vi "loadMT2FinalBin100Yld.vi"() -> ()   [LabVIEW 2012]
uses:
  <vilib>/addons/database/Auxilliary.llb/DB Tools Cursor Type.ctl
  <vilib>/addons/database/Connection.llb/DB Tools Open Connec (Path).vi
  <vilib>/addons/database/Connection.llb/Conn Execute.vi
  <vilib>/addons/database/Recordset.llb/Rec Fetch Recordset Data (R).vi
  <vilib>/addons/database/Recordset.llb/Rec Destroy - Connection.vi
  <vilib>/addons/database/_DB Variant To Data/Database Variant To Data.xnode
  <vilib>/addons/database/NI_Database_API.lvlib
panel:
  out "recordset data":variant[][](array[variant])
  out "data":string
  out "error out":errorcluster
  out "concatenated string":string
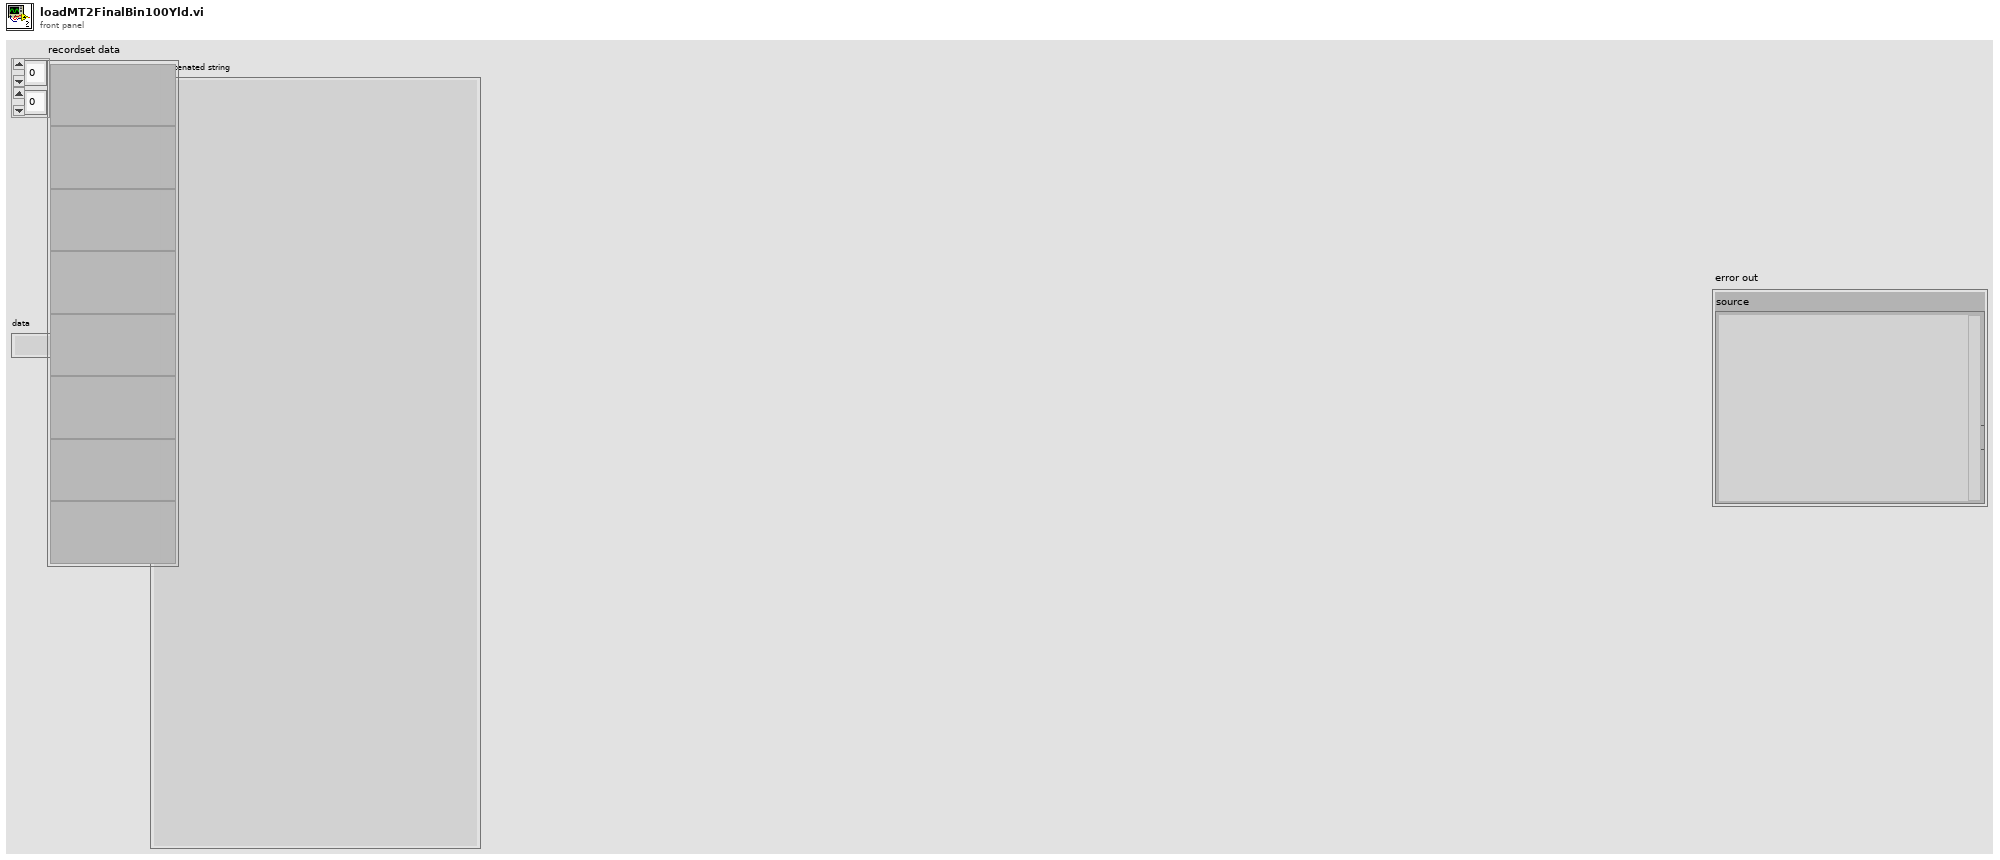
[diagram p1: front panel]
types:
  T1 = typedef "NI_Database_API.lvlib/DB Tools Cursor Type.ctl" = enum16{"forward-only", "keyset", "dynamic", "static"}
  T2 = typedef "NI_Database_API.lvlib/Conn ObjectReference.ctl" = refnum<k1>
  T3 = typedef "NI_Database_API.lvlib/Rec ObjectReference.ctl" = refnum<k1>
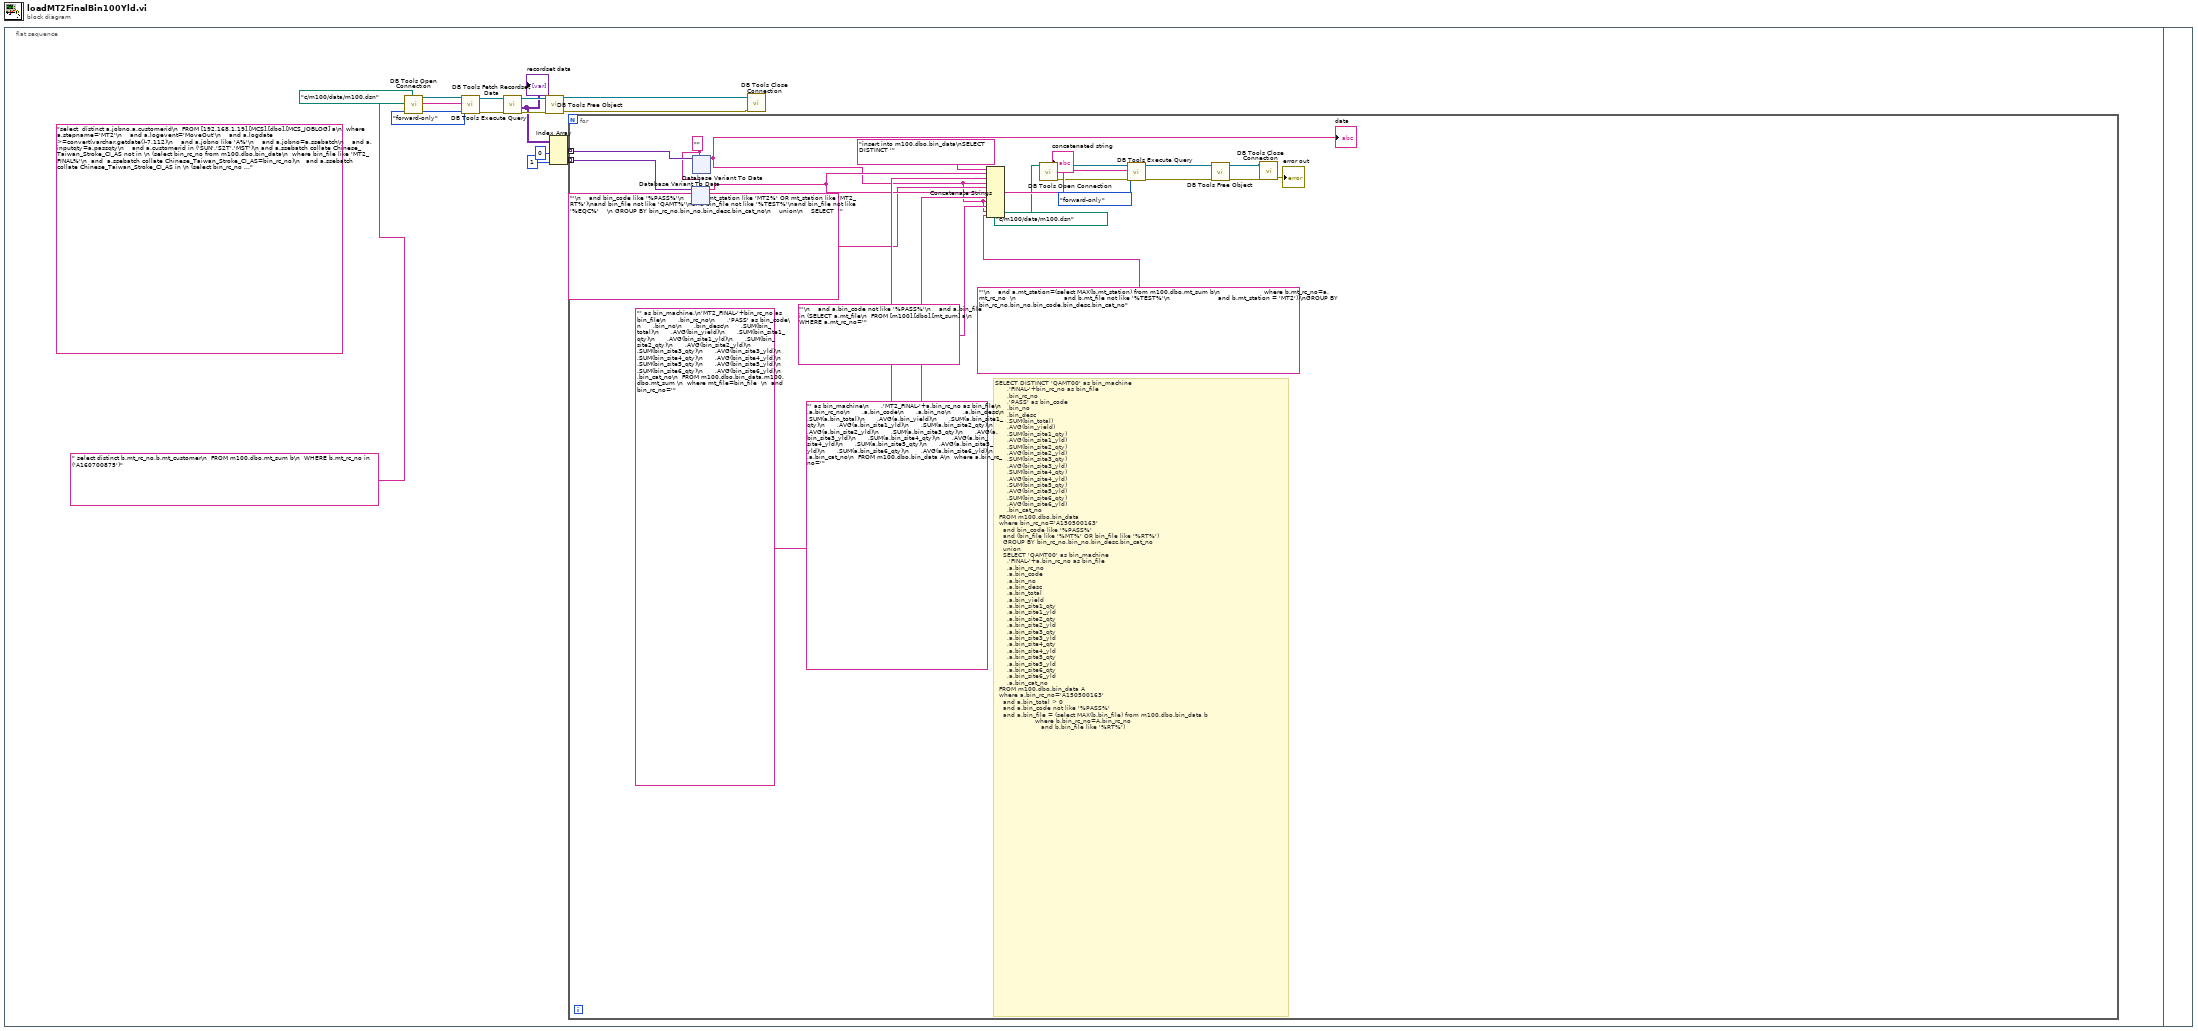
[diagram p0: block diagram]
diagram:
  n1 = flat-sequence {
    frame #0 {
      (unwired) "select  distinct a.jobno,a.customerid\n  FROM [192.168.1.19].[MCS].[dbo].[MCS_JOBLOG] a\n  where  a.stepname='MT2'\n    and a.logevent='MoveOut'\n    and a.logdate >=convert(varchar,getdate()-7,112)\n    and a.jobno like 'A%'\n    and a.jobno=a.ssebatch\n    and a.inputqty=a.passqty\n    and a.customerid in ('SUN','S2T','MST')\n and a.ssebatch collate Chinese_Taiwan_Stroke_CI_AS not in \n (select bin_rc_no from m100.dbo.bin_data\n  where bin_file like 'MT2_FINAL%'\n  and  a.ssebatch collate Chinese_Taiwan_Stroke_CI_AS=bin_rc_no)\n   and a.ssebatch collate Chinese_Taiwan_Stroke_CI_AS in \n (select bin_rc_no from m100.dbo.bin_data\n  where bin_file like '%MT2%'\n  and  a.ssebatch collate Chinese_Taiwan_Stroke_CI_AS=bin_rc_no)\n " ("SQL query")
      n2 = call-poly <vilib>:"DB Tools Open Connection.vi"("connection information"=path "c:/m100/data/m100.dsn") -> ("error out"=w13:errorcluster, "connection reference"=w16:T2)  [unwired: 7 in]
      n3 = call-poly <vilib>:"DB Tools Execute Query.vi"("error in (no error)"=w13, "cursor type"=DB_Tools_Cursor_Type."forward-only", "SQL query"=" select distinct b.mt_rc_no,b.mt_customer\n  FROM m100.dbo.mt_sum b\n  WHERE b.mt_rc_no in ('A160700875')", "connection reference"=w16) -> ("error out"=w12:errorcluster, "recordset reference"=w15:T3)  [unwired: 4 in]
      n4 = call-poly <vilib>:"DB Tools Fetch Recordset Data.vi"("error in (no error)"=w12, "recordset reference"=w15) -> ("error out"=w11:errorcluster, "recordset data"=w8:variant[][], "recordset reference out"=w14:T3)  [unwired: 3 in]
      "recordset data" <- w8
      n5 = call-poly <vilib>:"DB Tools Free Object.vi"("error in (no error)"=w11, "recordset reference"=w14) -> ("error out"=w4:errorcluster, "connection reference"=w5:T2)  [unwired: 8 in]
      n6 = Index Array(array=w8, index (col) #1=0 ("disabled index (col)"), index (col) #2=1 ("index (col)")) -> (element #1=w6:variant[], element #2=w2:variant[])  [unwired: 2 in]
      n7 = for {
        tunnel: w6 -> [w37] mode=indexing
        tunnel: w2 -> [w25] mode=indexing
        w24 = ""
        # "SELECT DISTINCT 'QAMT00' as bin_machine\n      ,'FINAL-'+bin_rc_no as bin_file\n      ,bin_rc_no\n      ,'PASS' as bin_code\n      ,bin_no\n      ,bin_desc\n      ,SUM(bin_total)\n      ,AVG(bin_yield)\n      ,SUM(bin_site1_qty)\n      ,AVG(bin_site1_yld)\n      ,SUM(bin_site2_qty)\n      ,AVG(bin_site2_yld)\n      ,SUM(bin_site3_qty)\n      ,AVG(bin_site3_yld)\n      ,SUM(bin_site4_qty)\n      ,AVG(bin_site4_yld)\n      ,SUM(bin_site5_qty)\n      ,AVG(bin_site5_yld)\n      ,SUM(bin_site6_qty)\n      ,AVG(bin_site6_yld)\n      ,bin_cat_no\n  FROM m100.dbo.bin_data\n  where bin_rc_no='A150500163'\n    and bin_code like '%PASS%'\n    and (bin_file like '%MT%' OR bin_file like '%RT%')\n    GROUP BY bin_rc_no,bin_no,bin_desc,bin_cat_no\n    union\n    SELECT 'QAMT00' as bin_machine\n      ,'FINAL-'+a.bin_rc_no as bin_file\n      ,a.bin_rc_no\n      ,a.bin_code\n      ,a.bin_no\n      ,a.bin_desc\n      ,a.bin_total\n      ,a.bin_yield\n      ,a.bin_site1_qty\n      ,a.bin_site1_yld\n      ,a.bin_site2_qty\n      ,a.bin_site2_yld\n      ,a.bin_site3_qty\n      ,a.bin_site3_yld\n      ,a.bin_site4_qty\n      ,a.bin_site4_yld\n      ,a.bin_site5_qty\n      ,a.bin_site5_yld\n      ,a.bin_site6_qty\n      ,a.bin_site6_yld\n      ,a.bin_cat_no\n  FROM m100.dbo.bin_data A\n  where a.bin_rc_no='A150500163'\n    and a.bin_total > 0\n    and a.bin_code not like '%PASS%'\n    and a.bin_file = (select MAX(b.bin_file) from m100.dbo.bin_data b\n                    where b.bin_rc_no=A.bin_rc_no\n                       and b.bin_file like '%RT%')"
        n8 = xnode "Database Variant To Data"("database variant"=w25, "type"=w24) -> ("data"=w20:string)  [unwired: 1 in, 1 out]
        n9 = xnode "Database Variant To Data"("database variant"=w37, "type"=w24) -> ("data"=w18:string)  [unwired: 1 in, 1 out]
        "data" <- w18
        n10 = Concatenate Strings("insert into m100.dbo.bin_data\nSELECT DISTINCT '" ("string"), w20, "' as bin_machine,\n'MT2_FINAL-'+bin_rc_no as bin_file\n      ,bin_rc_no\n      ,'PASS' as bin_code\n      ,bin_no\n      ,bin_desc\n      ,SUM(bin_total)\n      ,AVG(bin_yield)\n      ,SUM(bin_site1_qty)\n      ,AVG(bin_site1_yld)\n      ,SUM(bin_site2_qty)\n      ,AVG(bin_site2_yld)\n      ,SUM(bin_site3_qty)\n      ,AVG(bin_site3_yld)\n      ,SUM(bin_site4_qty)\n      ,AVG(bin_site4_yld)\n      ,SUM(bin_site5_qty)\n      ,AVG(bin_site5_yld)\n      ,SUM(bin_site6_qty)\n      ,AVG(bin_site6_yld)\n      ,bin_cat_no\n  FROM m100.dbo.bin_data,m100.dbo.mt_sum \n  where mt_file=bin_file  \n  and  bin_rc_no='" ("string"), w18, "'\n    and bin_code like '%PASS%'\n    and (mt_station like 'MT2%' OR mt_station like 'MT2_RT%')\nand bin_file not like 'QAMT%'\nand bin_file not like '%TEST%'\nand bin_file not like '%EQC%'    \n GROUP BY bin_rc_no,bin_no,bin_desc,bin_cat_no\n    union\n    SELECT  '" ("string"), w20, "' as bin_machine\n      ,'MT2_FINAL-'+a.bin_rc_no as bin_file\n      ,a.bin_rc_no\n      ,a.bin_code\n      ,a.bin_no\n      ,a.bin_desc\n       ,SUM(a.bin_total)\n      ,AVG(a.bin_yield)\n      ,SUM(a.bin_site1_qty)\n      ,AVG(a.bin_site1_yld)\n      ,SUM(a.bin_site2_qty)\n      ,AVG(a.bin_site2_yld)\n      ,SUM(a.bin_site3_qty)\n      ,AVG(a.bin_site3_yld)\n      ,SUM(a.bin_site4_qty)\n      ,AVG(a.bin_site4_yld)\n      ,SUM(a.bin_site5_qty)\n      ,AVG(a.bin_site5_yld)\n      ,SUM(a.bin_site6_qty)\n      ,AVG(a.bin_site6_yld)\n      ,a.bin_cat_no\n  FROM m100.dbo.bin_data A\n  where a.bin_rc_no='" ("string"), w18, "'\n    and a.bin_code not like '%PASS%'\n    and a.bin_file in (SELECT a.mt_file\n  FROM [m100].[dbo].[mt_sum] a\n  WHERE a.mt_rc_no='" ("string"), w18, "'\n    and a.mt_station=(select MAX(b.mt_station) from m100.dbo.mt_sum b\n                      where b.mt_rc_no=a.mt_rc_no  \n                        and b.mt_file not like '%TEST%'\n                        and b.mt_station = 'MT2'))\nGROUP BY bin_rc_no,bin_no,bin_code,bin_desc,bin_cat_no" ("string")) -> (w35:string)
        "concatenated string" <- w35
        n11 = call-poly <vilib>:"DB Tools Open Connection.vi"("connection information"=path "c:/m100/data/m100.dsn") -> ("error out"=w33:errorcluster, "connection reference"=w34:T2)  [unwired: 7 in]
        n12 = call-poly <vilib>:"DB Tools Execute Query.vi"("error in (no error)"=w33, "cursor type"=DB_Tools_Cursor_Type."forward-only", "SQL query"=w35, "connection reference"=w34) -> ("error out"=w27:errorcluster, "recordset reference"=w26:T3)  [unwired: 4 in]
        n13 = call-poly <vilib>:"DB Tools Free Object.vi"("error in (no error)"=w27, "recordset reference"=w26) -> ("error out"=w30:errorcluster, "connection reference"=w31:T2)  [unwired: 8 in]
        n14 = call <vilib>:"DB Tools Close Connection.vi"("error in (no error)"=w30, "connection reference"=w31) -> ("error out"=→"error out":errorcluster)  [unwired: 5 in]
      }
      n15 = call <vilib>:"DB Tools Close Connection.vi"("error in (no error)"=w4, "connection reference"=w5) -> ()  [unwired: 5 in, 1 out]
    }
    frame #1 {
    }
  }
